vi "Data_DisplayCfg.vi"(10 "路径":path) -> (1 "回读参数":T1, 2 "回放生效":bool)   [LabVIEW 2013]
panel:
  in  "取消":bool
  in  "确定":bool
  in  "刷新间隔(ms)":i32=100
  in  "单次回放点数":u64=10000
  in  "偏移点数":u64
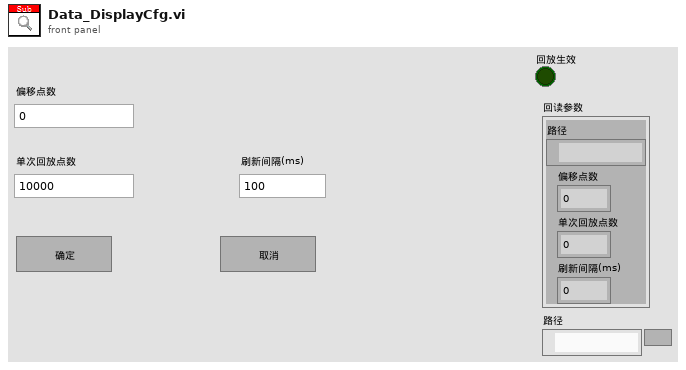
[diagram p1: front panel]
types:
  T1 = cluster{"路径":path, "偏移点数":u64, "单次回放点数":u64, "刷新间隔(ms)":i32}
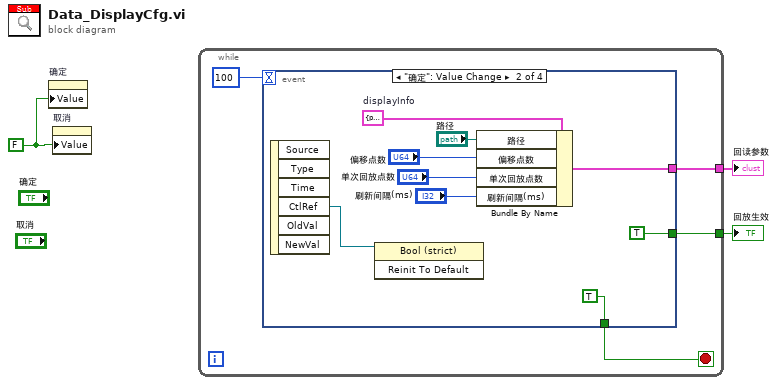
[diagram p0: block diagram]
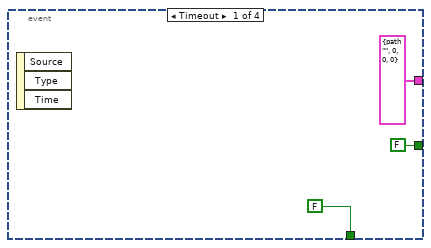
[diagram p2: hidden frame]
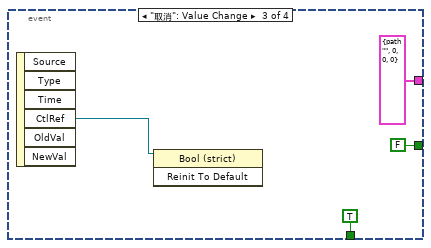
[diagram p3: hidden frame]
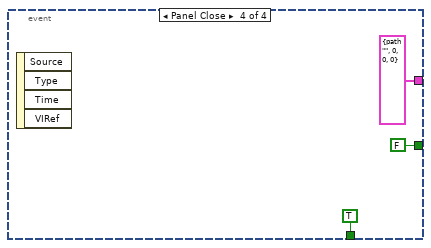
[diagram p4: hidden frame]
diagram:
  w1 = FALSE ("取消")
  n1 = property on="确定" class="Bool (strict)"("Value"=w1) -> ()  [unwired: 2 in, 2 out]
  n2 = property on="取消" class="Bool (strict)"("Value"=w1) -> ()  [unwired: 2 in, 2 out]
  n3 = while {
    tunnel: [w5] -> w3
    tunnel: [w4] -> w2
    stop <- w6 stop-if-true
    n4 = event shown="[1] \"确定\": Value Change" {
      selector: _ -> [_ _ _ _]
      dyn-events: _ -> [_ _ _ _]
      timeout: 100 -> [_ _ _ _]
      tunnel: [FALSE TRUE TRUE TRUE] -> w6
      tunnel: [T1 {"路径"=path "", "偏移点数"=0, "单次回放点数"=0, "刷新间隔(ms)"=0} ("displayInfo") w14 T1 {"路径"=path "", "偏移点数"=0, "单次回放点数"=0, "刷新间隔(ms)"=0} ("displayInfo") T1 {"路径"=path "", "偏移点数"=0, "单次回放点数"=0, "刷新间隔(ms)"=0} ("displayInfo")] -> w5
      tunnel: [FALSE TRUE FALSE FALSE] -> w4
      event Timeout {
        n5 = event-data() -> ()  [unwired: 1 in, 3 out]
      }
      event "确定": Value Change {
        w18 = T1 {"路径"=path "", "偏移点数"=0, "单次回放点数"=0, "刷新间隔(ms)"=0}  # displayInfo
        n6 = event-data() -> ("CtlRef"=w12:refnum<vi>)  [unwired: 1 in, 5 out]
        n7 = invoke class="Bool (strict)" method="Reinit To Default"(reference=w12) -> ()  [unwired: 2 in, 3 out]
        n8 = Bundle By Name(cluster=w18, "路径"="路径", "偏移点数"="偏移点数", "单次回放点数"="单次回放点数", "刷新间隔(ms)"="刷新间隔(ms)") -> (w14:T1)
      }
      event "取消": Value Change {
        n9 = event-data() -> ("CtlRef"=w20:refnum<vi>)  [unwired: 1 in, 5 out]
        n10 = invoke class="Bool (strict)" method="Reinit To Default"(reference=w20) -> ()  [unwired: 2 in, 3 out]
      }
      event Panel Close {
        n11 = event-data() -> ()  [unwired: 1 in, 4 out]
      }
    }
  }
  "回读参数" <- w3
  "回放生效" <- w2
